vi "test-nav-grid.vi"() -> ()   [LabVIEW 2019]
uses:
  <vilib>/Rock Robotics/WPI/ThirdParty/MJansen/PathPlanner/TypeDef/PathPlannerObstacleGrid.ctl
  <vilib>/Rock Robotics/WPI/ThirdParty/MJansen/PathPlanner/TypeDef/PathPlannerFinderGridPosition.ctl
  <vilib>/Rock Robotics/WPI/ThirdParty/MJansen/PathPlanner/PathPlanner24.lvlib
panel:
  out "Full Filename":string
  out "NavGridObstacles":T1[](array[typedef])
  out "PathPlanner_Grid":T2
  out "Field":cluster{"X":i32, "Y":i32}[](graph)
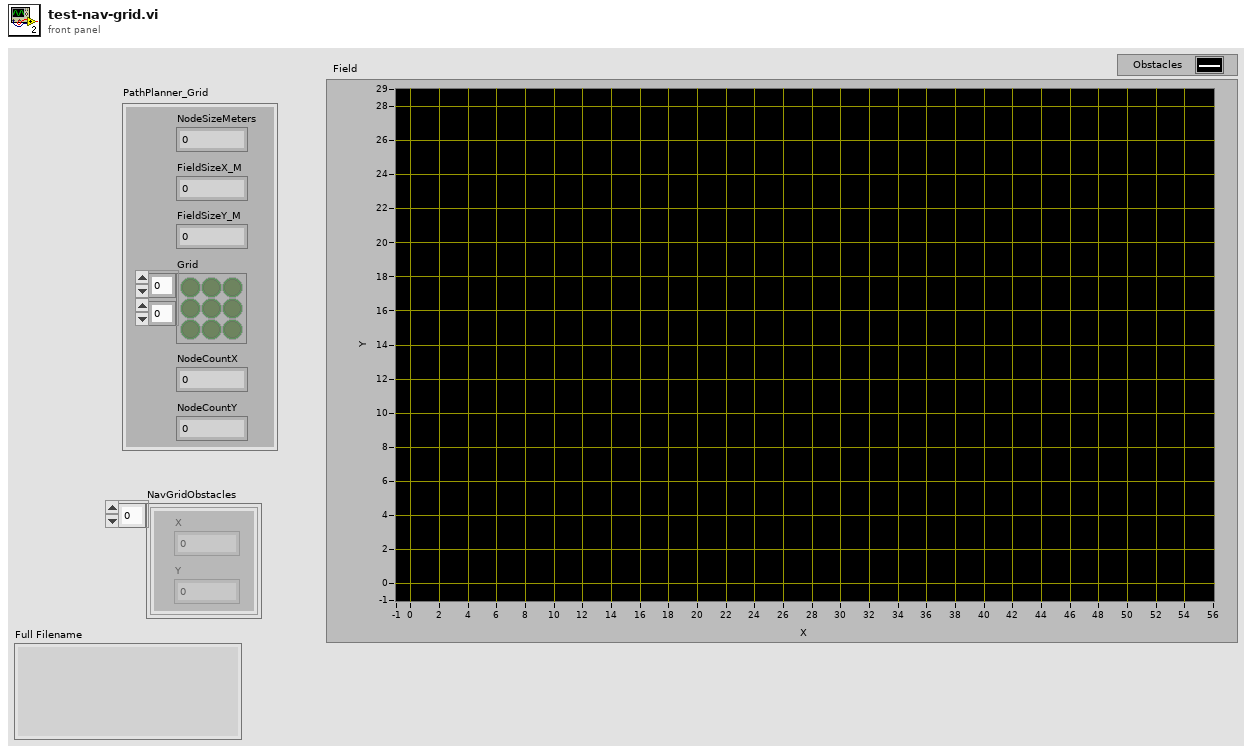
[diagram p1: front panel]
types:
  T1 = typedef "PathPlanner24.lvlib/PathPlannerFinderGridPosition.ctl" = cluster{"X":i32, "Y":i32}
  T2 = typedef "PathPlanner24.lvlib/PathPlannerObstacleGrid.ctl" = cluster{"NodeSizeMeters":dbl, "Grid":bool[][], "NodeCountX":i32, "NodeCountY":i32, "FieldSizeX_M":dbl, "FieldSizeY_M":dbl}
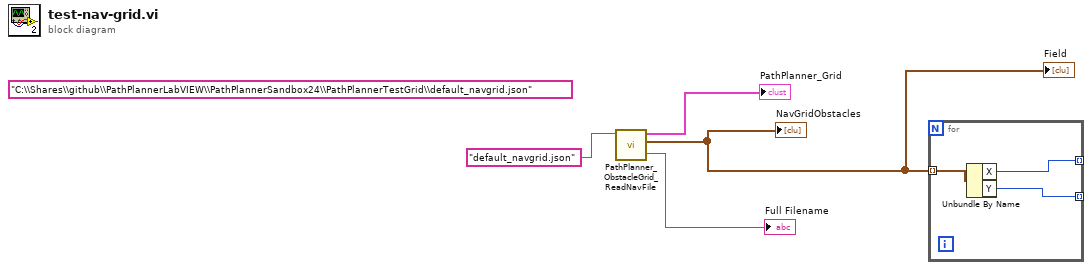
[diagram p0: block diagram]
diagram:
  (unwired) "C:\\Shares\\github\\PathPlannerLabVIEW\\PathPlannerSandbox24\\PathPlannerTestGrid\\default_navgrid.json" ("FileName")
  n1 = call <vilib>:"PathPlanner_ObstacleGrid_ReadNavFile.vi"("FileName"="default_navgrid.json") -> ("NavGridObstacles"=w2:T1[], "PathPlanner_Grid"=→"PathPlanner_Grid":T2, "Full Filename"=→"Full Filename":string)  [unwired: 7 in, 1 out]
  "Field" <- w2
  "NavGridObstacles" <- w2
  n2 = for {
    tunnel: w2 -> [w7] mode=indexing
    tunnel: [w6] -> _ mode=indexing
    tunnel: [w5] -> _ mode=indexing
    n3 = Unbundle By Name(w7) -> ("X"=w6:i32, "Y"=w5:i32)
  }
